vi "Stop Core.vi"(10 "final error code":i32, 11 "Inspection Statemachine in":refnum<class "Inspection Statemachine.lvclass">) -> (3 "Inspection Statemachine out":refnum<class "Inspection Statemachine.lvclass">)   [LabVIEW 2019, in "Inspection Statemachine.lvclass"]
doc: "(<B>Filename</B>: Actor Framework.lvlib:Actor.lvclass:Stop Core.vi)\n\nDefines what the actor does before it stops. Use the <B>final error code</B> input to determine whether the actor shut down in response to an error.\n\nBy default, this method does nothing. A descendant class may override it to define behavior, such as shutting down any processes the actor initiated in its override of the Actor Core method."
uses:
  Inspection Statemachine.lvclass
  <vilib>/ActorFramework/Actor/Actor.lvclass
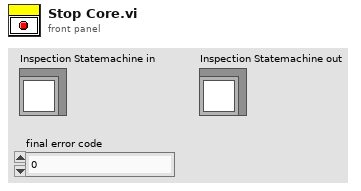
[diagram p1: front panel]
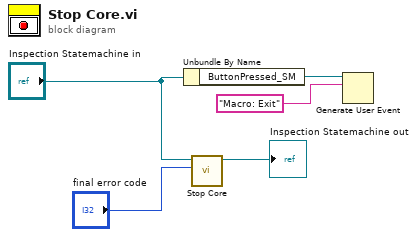
[diagram p0: block diagram]
diagram:
  n1 = Unbundle By Name("Inspection Statemachine in") -> ("ButtonPressed_SM"=w2:refnum<user-event>)
  n2 = call-parent "Stop Core.vi"("final error code"="final error code", "Actor in"="Inspection Statemachine in") -> ("Actor out"=→"Inspection Statemachine out":refnum<class "Inspection Statemachine.lvclass">)  [unwired: 9 in]
  n3 = Generate User Event(user event=w2, event data cluster="Macro: Exit" ("event data")) -> ()  [unwired: 2 in, 2 out]
